vi "3_1_Objects_Detection(Deploy)(File).vi"() -> ()   [LabVIEW 2020]
doc: "This example demonstrates the process of loading pretrained model for objects detection and running for inference/prediction.\nRequirements: 1. Deep Learning Toolkit for LabVIEW (v3.0 and above).\n 2. NI Vision Development Module.\n 3. Trained model generated during training."
uses:
  <vilib>/Ngene/Deep Learning Toolkit/Toolkit/NN_Network/Controls/NN_Device.ctl
  <vilib>/Ngene/Deep Learning Toolkit/Toolkit/NN_Data/API/NN_Dims(C,H,W).ctl
  <vilib>/Ngene/Deep Learning Toolkit/Toolkit/NN_Network/Controls/NN_Save_Before_Destroy_Options.ctl
  db58ee50-833d-44de-af7a-1cdf2c93578f.vi
  a19d14a2-56a0-482f-a821-023949621d05.vi
  <vilib>/Utility/High Resolution Relative Seconds.vi
  <vilib>/Ngene/Deep Learning Toolkit/Toolkit/Utils/Vision/Coords_Rect2PolyLine.vi
  <vilib>/Ngene/Deep Learning Toolkit/Toolkit/NN_Network/API/NN_Set_Input/3D/NN_Set_Input(3D_SGL_idx).vi
  <vilib>/Ngene/Deep Learning Toolkit/Toolkit/Deep_Learning_Toolkit_by_Ngene.lvlib
  <vilib>/ptbypt/NI_PtbyPt.lvlib
panel:
  out "Dims_In":T1={"C"=3, "H"=512, "W"=910}
  out "Inference Time":dbl=0.37406049000055647 format="%#_2p"
  out "Sample Path":path=path "D:/Ngene/GitHub/deepltk_examples/3_Image_Processing/33_Object_Detection/Dataset/Orig/Test/Images/114.png"
  in  "Select Sample":i32=5 min=0 max=73 step=1
  in  "Dataset (Images)":path=path "D:/Ngene/GitHub/deepltk_examples/3_Image_Processing/33_Object_Detection/Dataset/0_Orig/Test/Images"
  in  "NN_Device":T2
  out "FPS":dbl=2.673364406913204 format="%#_2p"
  out "Display":T3(plugin-control)
  in  "Confidence_Thresh":sgl=0.482
  in  "IOU_Thresh(NMS)":sgl=0.43
  in  "Stop":bool
  in  "Model Weights":path=path "D:/Ngene/GitHub/deepltk_examples/3_Image_Processing/33_Object_Detection/Trained Model/512x910_mAP_0.998/Obj_Det_Example_weights_25_06_09__13_45_53.bin"
  in  "Model Topology (CFG)":path=path "D:/Ngene/GitHub/deepltk_examples/3_Image_Processing/33_Object_Detection/Trained Model/512x910_mAP_0.998/Obj_Det_Example_net_cfg_25_06_09__13_45_53.cfg"
  # "Overview: This example demonstrates the process of deploying an object detection model for inference.\nRequirements: \n1. Deep Learning Toolkit for LabVIEW.\n2. NI Vision Development Module.\n3. Trained model generated during training.\nInstructions:\n1. Provide \"Model Topology\" and \"Model Weights\" generated after training in \"1_Objects_Detection(Train).vi\".\n2. Provide path to the folder with test images at \"Dataset (Images)\" . \n3. Run the VI.\n4. Change \"Select Sample\" value to select different image samples from the datset.\n5. Press \"Stop\" button to stop the VI.\n\nMore Examples:  https://github.com/ngenehub/deepltk_examples"
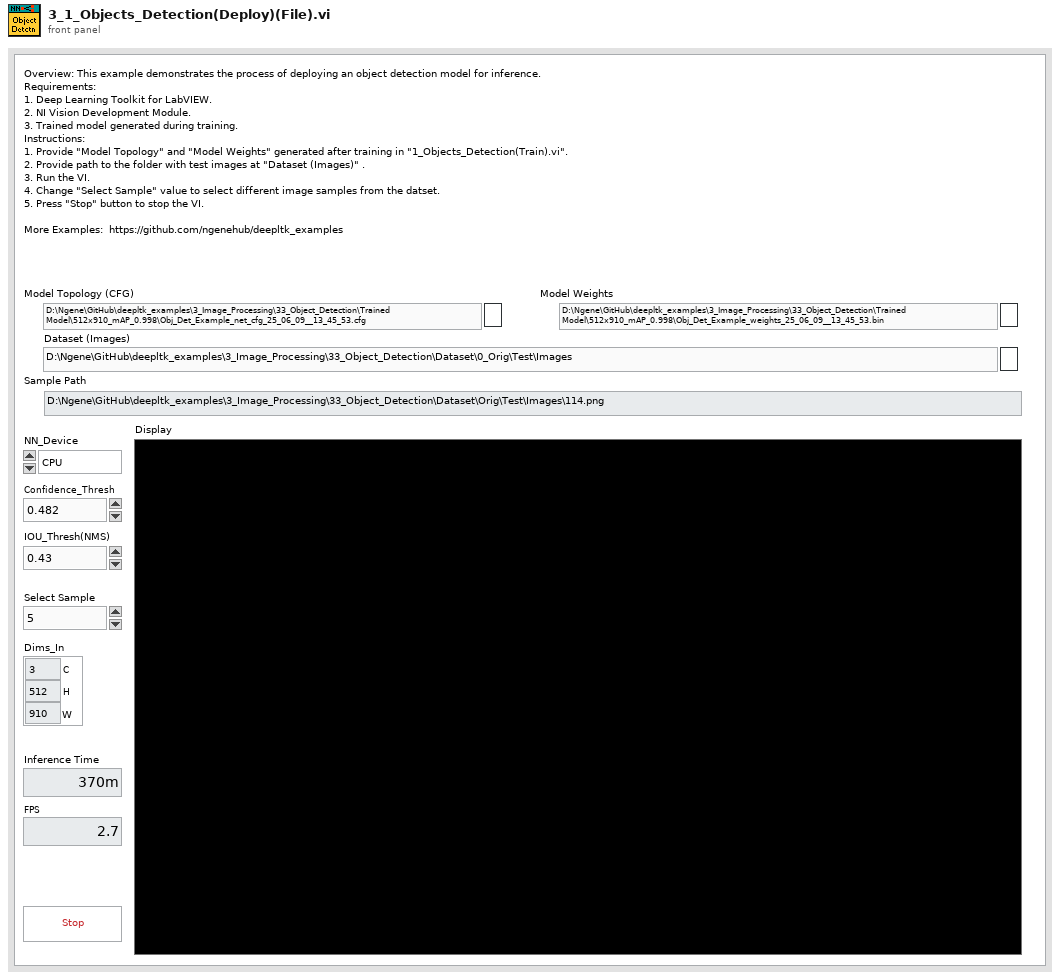
[diagram p1: front panel]
types:
  T1 = typedef "Deep_Learning_Toolkit_by_Ngene.lvlib/NN_Dims(C,H,W).ctl" = cluster{"C":i32, "H":i32, "W":i32}
  T2 = typedef "Deep_Learning_Toolkit_by_Ngene.lvlib/NN_Device.ctl" = enum16{"CPU", "GPU"}
  T3 = typedef "IMAQ Image.ctl" = refnum<image>
  T4 = typedef "Deep_Learning_Toolkit_by_Ngene.lvlib/NN_Save_Before_Destroy_Options.ctl" = cluster{"CFG?":bool, "Weights?":bool, "Render?":bool}
  T5 = typedef "Deep_Learning_Toolkit_by_Ngene.lvlib/NN_Config_Params.ctl" = cluster{"Name":string, "mBatch":i32, "NN_Train_Params":T6, "LR_Decay_Policy":T9, "Labels":string[], "Loss":T11, "Max_WS_Size(B)":i64, "DryRun?":bool}
  T6 = typedef "Deep_Learning_Toolkit_by_Ngene.lvlib/NN_Train_Params.ctl" = cluster{"Optimizer":T7, "Beta_1":sgl, "Beta_2":sgl, "Weight Decay(L1)":sgl, "Weight Decay(L2)":sgl, "Data_Sampling":T8}
  T7 = typedef "Deep_Learning_Toolkit_by_Ngene.lvlib/NN_Train_Optimizer.ctl" = enum16{"SGD", "Adam", "Adagrad", "Adadelta", "RMSProp", "Nesterov"}
  T8 = typedef "Deep_Learning_Toolkit_by_Ngene.lvlib/NN_Train_Data_Sampling.ctl" = enum16{"Random", "Sequential"}
  T9 = typedef "Deep_Learning_Toolkit_by_Ngene.lvlib/NN_LR_Policy_Cfg.ctl" = cluster{"Policy_Type":T10, "LR0":dbl, "k":sgl, "WarmUp_Policy":enum16{"Step", "Ramp"}, "WarmUp_Iter":i32, "WarmUp_Ratio":sgl}
  T10 = typedef "Deep_Learning_Toolkit_by_Ngene.lvlib/NN_LR_Policy_Type.ctl" = enum16{"Manual", "Step", "Exp", "1/t"}
  T11 = typedef "Deep_Learning_Toolkit_by_Ngene.lvlib/NN_Loss_Config_Params.ctl" = cluster{"Loss_Type":T12, "Loss_Conf_Params":variant}
  T12 = typedef "Deep_Learning_Toolkit_by_Ngene.lvlib/NN_Loss_Type.ctl" = enum16{"None", "MSE", "CrossEntropy", "YOLO_v2", "YOLO_v4"}
  T13 = typedef "Deep_Learning_Toolkit_by_Ngene.lvlib/NN_Layer_Config_Params.ctl" = cluster{"Layer_Type":T14, "Layer_Conf_Params":variant, "Input Layers":string[]}
  T14 = typedef "Deep_Learning_Toolkit_by_Ngene.lvlib/NN_Layer_Type.ctl" = enum16{"Input1D", "Input3D", "Conv1D", "Conv2D", "Conv2D_Adv", "MaxPool", "AvgPool", "UpSample", "DropOut3D", "ShortCut", "Concat", "SoftMax3D", "FC", "DropOut", "Softmax", "Flatten", "YOLO_v2", "YOLO_v4", "Activation", "BatchNormalization", "LayerNormalization", "Scale", "Unsupported"}
  T15 = typedef "Deep_Learning_Toolkit_by_Ngene.lvlib/NN.ctl" = cluster{"Name":string, "No of Layers":i32, "mBatch":i32, "Layers":T16[], "Dimty":T17, "Dims_In":T1, "Dims_Out":T1, "Working_Dir":path, "Train?":bool, "Train_Params":T6, "LR_Update_Policy":T9, "Session Data":T18, "Ground_truth":T19, "NNg_hdls":T20, "NN_Device":T2, "GPU Id":i32, "Labels":string[], "Loss_Type":T12, "Loss_Cfg_Prms":variant, "NNG_WS":T21, "DryRun?":bool}
  T16 = typedef "Deep_Learning_Toolkit_by_Ngene.lvlib/NN_Layer_ref.ctl" = refnum<file>
  T17 = typedef "Deep_Learning_Toolkit_by_Ngene.lvlib/NN_In_Out_Dim-ty.ctl" = enum8{"In1D_Out1D", "In3D_Out1D", "In3D_Out3D", "In3D_OutBBox"}
  T18 = typedef "Deep_Learning_Toolkit_by_Ngene.lvlib/NN_Train_Session_Data.ctl" = cluster{"Epochs":sgl, "Tot_Iter":i32, "LR":sgl, "LR_iter":i32}
  T19 = typedef "Deep_Learning_Toolkit_by_Ngene.lvlib/NN_Ground_truth.ctl" = cluster{"Y":variant}
  T20 = typedef "Deep_Learning_Toolkit_by_Ngene.lvlib/nng_cuda_handles.ctl" = cluster{"cudnn":u64, "cublas":u64, "stream":u64, "curand":u64}
  T21 = typedef "Deep_Learning_Toolkit_by_Ngene.lvlib/NNG_WS.ctl" = cluster{"NNG_WS_Mem":T22, "Max_WS_Size":i64}
  T22 = typedef "Deep_Learning_Toolkit_by_Ngene.lvlib/NNg_WS_Mem_DVR.ctl" = refnum<data-value>
  T23 = typedef "Deep_Learning_Toolkit_by_Ngene.lvlib/NN_Layer.ctl" = cluster{"Name":string, "Layer_Data":T24, "Layer_Type":T14, "Dims_In":T1, "Layers_In":T16[], "Dims_Out":T1, "Layers_Out":T16[], "Metrics":T25, "GPU_Data":T26, "mBatch":i32, "NN_Device":T2, "NNg_hdls":T20, "Train?":bool, "Dimty":T27, "RecptField":T28, "Idx":i32}
  T24 = typedef "Deep_Learning_Toolkit_by_Ngene.lvlib/NN_Layer_Data_Refnum.ctl" = refnum<file>
  T25 = typedef "Deep_Learning_Toolkit_by_Ngene.lvlib/NN_Layer_Metrics.ctl" = cluster{"Data":dbl, "Params":dbl, "Ops":dbl}
  T26 = typedef "Deep_Learning_Toolkit_by_Ngene.lvlib/NNg_Layer_Data_Refnum.ctl" = refnum<file>
  T27 = typedef "Deep_Learning_Toolkit_by_Ngene.lvlib/NN_Layer_Dimty.ctl" = enum16{"1D", "3D"}
  T28 = typedef "Deep_Learning_Toolkit_by_Ngene.lvlib/NN_Layer_RF_State.ctl" = cluster{"Dims":T29, "J":T29}
  T29 = typedef "Deep_Learning_Toolkit_by_Ngene.lvlib/NN_Dims(V,H).ctl" = cluster{"V":i32, "H":i32}
  T30 = typedef "Deep_Learning_Toolkit_by_Ngene.lvlib/NN_BBox_Detection.ctl" = cluster{"Class":i32, "Conf Level":sgl, "BBox":T31}
  T31 = typedef "Deep_Learning_Toolkit_by_Ngene.lvlib/NN_BBox.ctl" = cluster{"x":sgl, "y":sgl, "w":sgl, "h":sgl}
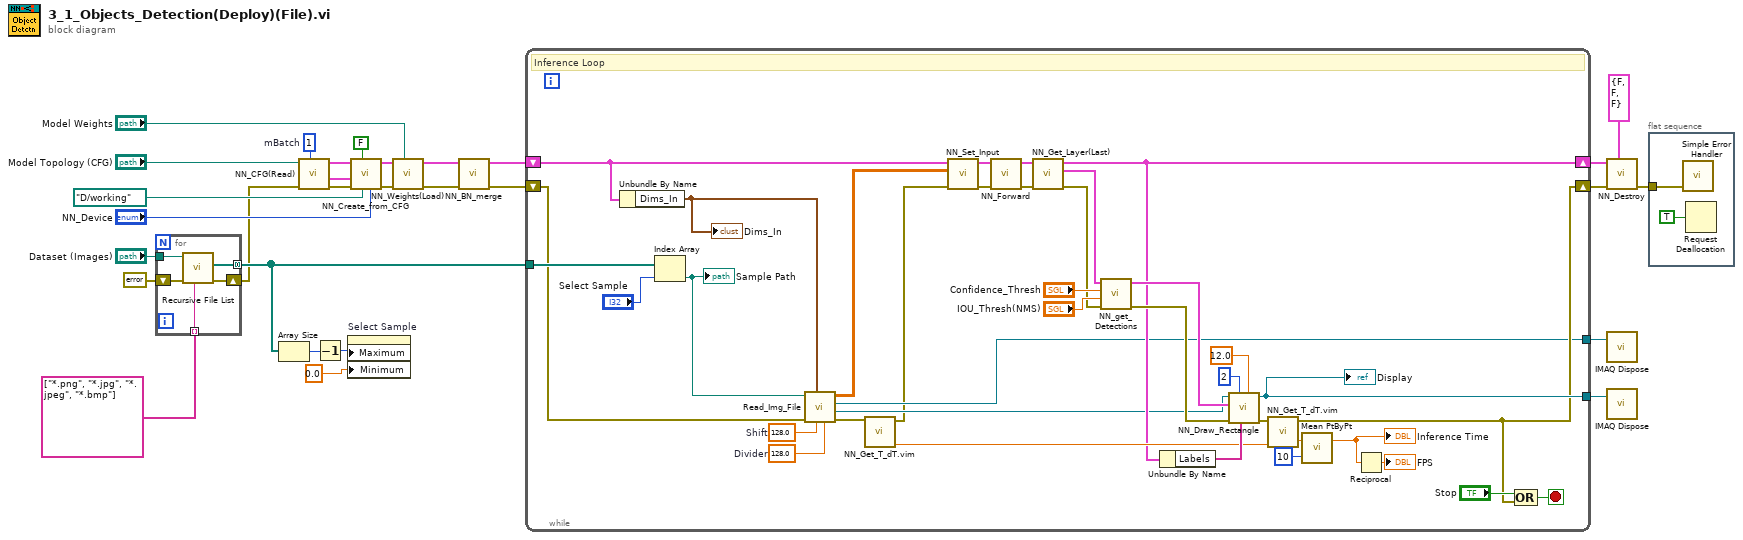
[diagram p0: block diagram]
diagram:
  w13 = 1  # mBatch
  n1 = for {
    tunnel: "Dataset (Images)" -> [w34]
    tunnel: string[] ["*.png", "*.jpg", "*.jpeg", "*.bmp"] ("pattern") -> [w33] mode=indexing
    tunnel: [w32] -> w9 mode=concatenating
    shift-right: [w30] -> w7
    shift-left: errorcluster {"status"=FALSE, "code"=0, "source"=""} ("error out") -> [w31]
    n2 = call <vilib>:"Recursive File List.vi"("pattern"=w33, "error in (no error)"=w31, "Folder Path"=w34) -> ("error out"=w30:errorcluster, "All Files in Dir"=w32:path[])  [unwired: 4 in, 3 out]
  }
  n3 = Array Size(array=w9) -> (size(s)=w10:i32)
  n4 = call <vilib>:"NN_CFG(Read).vi"("mBatch"=w13, "error in (no error)"=w7, "CFG file path"="Model Topology (CFG)") -> ("error out"=w27:errorcluster, "Net_Cfg"=w12:T5, "Layer_Cfg"=w28:T13[])  [unwired: 6 in]
  n5 = Decrement(x=w10) -> (x-1=w8:i32)
  n6 = property on="Select Sample" class="DigNum (strict)"("Maximum"=w8, "Minimum"=0.0 ("Data Entry Limits:Minimum")) -> ()  [unwired: 2 in, 2 out]
  n7 = call <vilib>:"NN_Create_from_CFG.vi"("NN_Device"="NN_Device", "Working Dir"=path "D:/working", "Train? (false)"=FALSE ("Train?"), "error in (no error)"=w27, "Net_Cfg"=w12, "Layer_Cfg"=w28) -> ("error out"=w26:errorcluster, "NN out"=w24:T15)  [unwired: 4 in]
  n8 = call <vilib>:"NN_Weights(Load).vi"("Weight File Path"="Model Weights", "error in (no error)"=w26, "NN in"=w24) -> ("error out"=w6:errorcluster, "NN out"=w2:T15)  [unwired: 7 in]
  n9 = call <vilib>:"NN_BN_merge.vi"("error in (no error)"=w6, "NN in"=w2) -> ("error out"=w3:errorcluster, "NN out"=w1:T15)  [unwired: 8 in]
  n10 = while {
    shift-right: [w45] -> w22
    shift-left: w1 -> [w47]
    tunnel: [w55] -> w23
    tunnel: w9 -> [w65]
    shift-right: [w51] -> w15
    shift-left: w3 -> [w63]
    tunnel: [w41] -> w4
    stop <- w70 stop-if-true
    w42 = sgl 128.0  # Divider
    w43 = sgl 128.0  # Shift
    # "Inference Loop"
    n11 = Unbundle By Name(w47) -> ("Dims_In"=w37:T1)
    "Dims_In" <- w37
    n12 = Index Array(array=w65, index="Select Sample") -> (element=w54:path)
    "Sample Path" <- w54
    n13 = call "Read_Img_File.vi"("Divider"=w42, "Shift"=w43, "Dims(C,H,W)"=w37, "error in (no error)"=w63, "Path"=w54) -> ("error out"=w53:errorcluster, "Image(Orig)"=w40:T3, "Image(Resampled)"=w41:T3, "Image Data"=w38:sgl[][][])  [unwired: 3 in]
    n14 = call "NN_Get_T_dT.vim"("error in"=w53) -> ("T_out"=w46:dbl, "error out"=w39:errorcluster)  [unwired: 6 in, 1 out]
    n15 = call-poly <vilib>:"NN_Set_Input.vi"("error in (no error)"=w39, "Data_In(3D_SGL)"=w38, "NN in"=w47) -> ("error out"=w58:errorcluster, "NN out"=w59:T15)  [unwired: 7 in]
    n16 = call <vilib>:"NN_Forward.vi"("error in (no error)"=w58, "NN in"=w59) -> ("error out"=w60:errorcluster, "NN out"=w61:T15)  [unwired: 6 in, 2 out]
    n17 = call <vilib>:"NN_Get_Layer(Last).vi"("error in (no error)"=w60, "NN in"=w61) -> ("error out"=w62:errorcluster, "Last_Layer"=w44:T23, "NN out"=w45:T15)  [unwired: 6 in, 1 out]
    n18 = call <vilib>:"NN_get_Detections.vi"("error in"=w62, "IOU_Thrsh"="IOU_Thresh(NMS)", "Confidence_Thrsh"="Confidence_Thresh", "YOLO_Layer"=w44) -> ("error out"=w56:errorcluster, "Detections"=w57:T30[])  [unwired: 6 in]
    n19 = Unbundle By Name(w45) -> ("Labels"=w48:string[])
    n20 = call "NN_Draw_Rectangle.vi"("font_size"=sgl 12.0 ("fontsize"), "Labels"=w48, "Border_Width"=u32 2, "error in (no error)"=w56, "Draw_Boxes"=w57, "Img in"=w40) -> ("error out"=w52:errorcluster, "Img out"=w55:T3)  [unwired: 4 in]
    "Display" <- w55
    n21 = call "NN_Get_T_dT.vim"("T_in"=w46, "error in"=w52) -> ("error out"=w51:errorcluster, "dT"=w50:dbl)  [unwired: 5 in, 1 out]
    n22 = call <vilib>:"Mean PtByPt.vi"("x"=w50, "sample length"=10) -> ("mean"=w36:dbl)  [unwired: 2 in, 1 out]
    "Inference Time" <- w36
    n23 = Reciprocal(x=w36) -> (1/x=→"FPS":dbl)
    n24 = Compound Arithmetic op=OR("Stop", w51) -> (w70:bool)
  }
  n25 = call <vilib>:"NN_Destroy.vi"("Save (T, T, T)"=T4 {"CFG?"=FALSE, "Weights?"=FALSE, "Render?"=FALSE} ("Save_Config"), "error in (no error)"=w15, "NN in"=w22) -> ("error out"=w14:errorcluster)  [unwired: 7 in, 1 out]
  n26 = call "IMAQ Dispose"("Image"=w4) -> ()  [unwired: 5 in, 1 out]
  n27 = call "IMAQ Dispose"("Image"=w23) -> ()  [unwired: 5 in, 1 out]
  n28 = flat-sequence {
    tunnel: w14 -> [w72]
    frame #0 {
      n29 = call <vilib>:"Simple Error Handler.vi"("error in (no error)"=w72) -> ()  [unwired: 4 in, 5 out]
      n30 = Request Deallocation(TRUE ("flag")) -> ()
    }
  }
